vi "Temp ID FG.vi"(11 "Entity":refnum<class "Entity.lvclass">) -> (2 "New ID":T1)   [LabVIEW 2020, in "Conditum.lvlib" / "Entity.lvclass"]
uses:
  Entity.lvclass
  <vilib>/Utility/miscctls.llb/LVMapReplaceAction.ctl
  Entity ID.ctl
  Conditum.lvlib
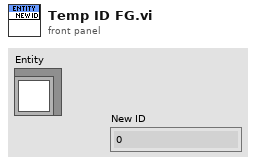
[diagram p1: front panel]
types:
  T1 = typedef "Conditum.lvlib/Entity ID.ctl" = i64
  T2 = typedef "LVMapReplaceAction.ctl" = enum32{"Modify Entry only if found", "Add or Modify Entry", "Delete Entry"}
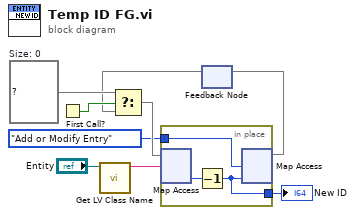
[diagram p0: block diagram]
diagram:
  w8 = map{string, T1} {}  # Size: 0
  n1 = First Call?() -> (First Call?: T/F=w9:bool)
  n2 = call <vilib>:"Get LV Class Name.vi"("object"="Entity") -> ("class name"=w4:string)  [unwired: 9 in, 1 out]
  n3 = feedback #1() -> (w7:map{string, T1})  [unwired: 1 in]
  n4 = Select(t=w8, s=w9, f=w7) -> (s? t:f=w5:map{string, T1})
  n5 = in-place {
    in-place-border: [w11] -> w1
    in-place-border: LVMapReplaceAction."Add or Modify Entry" ("action") -> [w10]
    n6 = in-place-map #2(w5, w4) -> (w12:T1)  [unwired: 1 in, 1 out]
    n7 = Decrement(x=w12) -> (x-1=w11:T1)
    n8 = in-place-map #2(w11, w10) -> (w2:map{string, T1})  [unwired: 2 out]
  }
  "New ID" <- w1
  n9 = feedback-in #1(w2) -> ()
